vi "Auto Detect_Programming Mode_List Slots.vi"(5 "Password":string, 7 "User Name":string, 8 "error in (no error)":errorcluster, 11 "serverName In":string) -> (0 "error out":errorcluster, 1 "Resources out":refnum<k20>[](array[refnum]), 2 "Session out":refnum<k21>, 3 "Refnum out":refnum<k20>)   [LabVIEW 2017, in "Scan Engine Custom Device.lvlib"]
doc: "List slots (supporting property \"Slot Programming Mode\") populated."
uses:
  Scan Engine Custom Device.lvlib
  <vilib>/nisyscfg/Filter Mode.ctl
  <vilib>/nisyscfg/nisyscfg.lvlib
  <resource>/objmgr/niflexrioatomicsae.rc
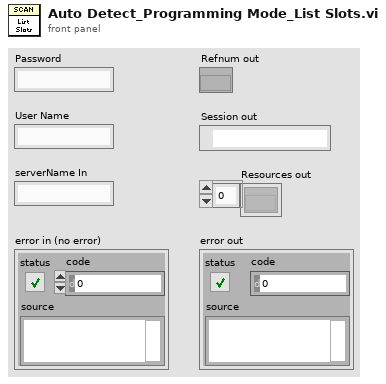
[diagram p1: front panel]
types:
  T1 = typedef "nisyscfg.lvlib/Filter Mode.ctl" = i32
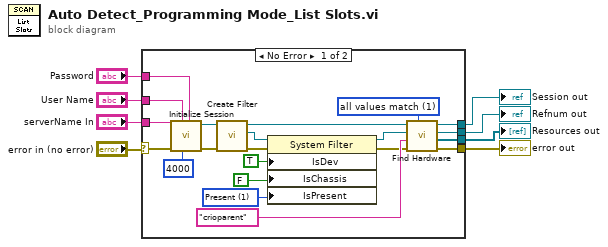
[diagram p0: block diagram]
diagram:
  n1 = case shown="No Error" "error in (no error)" {
    selector: "error in (no error)" -> [w9 w30]
    tunnel: [w29 _] -> w8
    tunnel: [w28 w30] -> w7
    tunnel: [w14 _] -> w6
    tunnel: [w13 _] -> w5
    tunnel: "Password" -> [w12 _]
    tunnel: "User Name" -> [w11 _]
    tunnel: "serverName In" -> [w10 _]
    frame No Error {
      w26 = 1 items=["Initializing"=-2, "Unknown"=-1, "Not Present"=0, "Present"=1] ("Devices & Chassis:Is Present")
      w22 = T1 1 items=["all values match"=1, "any value matches"=2, "values do not match"=3, "all properties exist"=4] ("filter mode (all values match)")
      n2 = call <vilib>:"Initialize Session.vi"("Password"=w12, "Connect Timeout (4000 ms)"=u32 4000, "User Name"=w11, "error in (no error)"=w9, "Target (localhost)"=w10) -> ("error out"=w20:errorcluster, "Session out"=w17:refnum<k21>)  [unwired: 5 in]
      n3 = call <vilib>:"Create Filter.vi"("error in (no error)"=w20, "Session in"=w17) -> ("error out"=w15:errorcluster, "Filter out"=w16:refnum<k20>, "Session out"=w18:refnum<k21>)  [unwired: 7 in]
      n4 = property class="System Filter"(reference=w16, error in=w15, "IsDev"=TRUE ("Is Device"), "IsChassis"=FALSE ("Is Chassis"), "IsPresent"=w26) -> (reference out=w21:refnum<k20>, error out=w19:errorcluster)
      n5 = call <vilib>:"Find Hardware.vi"("Filter Mode (all values match)"=w22, "error in (no error)"=w19, "Experts"="crioparent" ("Expert Info:Expert Name"), "Filter in"=w21, "Session in"=w18) -> ("error out"=w28:errorcluster, "Resources out"=w13:refnum<k20>[], "Filter out"=w29:refnum<k20>, "Session out"=w14:refnum<k21>)  [unwired: 3 out]
    }
    frame Error {
    }
  }
  "Refnum out" <- w8
  "error out" <- w7
  "Session out" <- w6
  "Resources out" <- w5
